vi "Joystick Deadband.vi"(6 "Z Deadband":dbl, 7 "X Y Deadband":dbl, 9 "Z":dbl, 10 "Y":dbl, 11 "X":dbl) -> (1 "Z Out":dbl, 2 "Y Out":dbl, 3 "X Out":dbl)   [LabVIEW 2018]
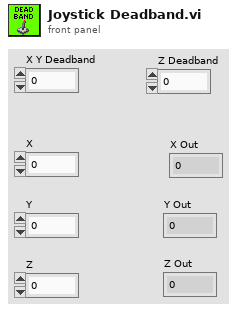
[diagram p1: front panel]
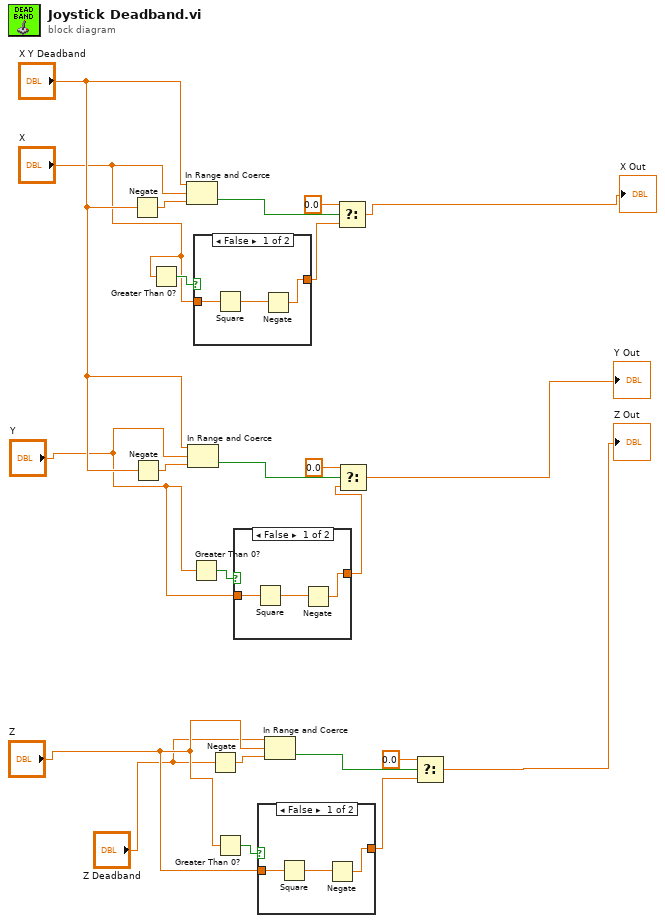
[diagram p0: block diagram]
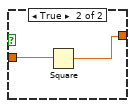
[diagram p2: hidden frame]
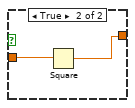
[diagram p3: hidden frame]
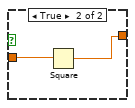
[diagram p4: hidden frame]
diagram:
  n1 = Negate(x="X Y Deadband") -> (-x=w23:dbl)
  n2 = Negate(x="X Y Deadband") -> (-x=w20:dbl)
  n3 = Greater Than 0?(x="X") -> (x > 0?=w10:bool)
  n4 = In Range and Coerce(upper limit="X Y Deadband", x="X", lower limit=w23) -> (In Range?=w22:bool)  [unwired: 1 out]
  n5 = In Range and Coerce(upper limit="X Y Deadband", x="Y", lower limit=w20) -> (In Range?=w19:bool)  [unwired: 1 out]
  n6 = Greater Than 0?(x="Y") -> (x > 0?=w8:bool)
  n7 = case shown="False" w10 {
    tunnel: [w24 w27] -> w11
    tunnel: "X" -> [w26 w28]
    frame False {
      n8 = Square(x=w26) -> (x^2=w25:dbl)
      n9 = Negate(x=w25) -> (-x=w24:dbl)
    }
    frame True {
      n10 = Square(x=w28) -> (x^2=w27:dbl)
    }
  }
  n11 = Negate(x="Z Deadband") -> (-x=w14:dbl)
  n12 = Greater Than 0?(x="Z") -> (x > 0?=w5:bool)
  n13 = case shown="False" w8 {
    tunnel: [w29 w32] -> w6
    tunnel: "Y" -> [w31 w33]
    frame False {
      n14 = Square(x=w31) -> (x^2=w30:dbl)
      n15 = Negate(x=w30) -> (-x=w29:dbl)
    }
    frame True {
      n16 = Square(x=w33) -> (x^2=w32:dbl)
    }
  }
  n17 = case shown="False" w5 {
    tunnel: [w34 w37] -> w4
    tunnel: "Z" -> [w36 w38]
    frame False {
      n18 = Square(x=w36) -> (x^2=w35:dbl)
      n19 = Negate(x=w35) -> (-x=w34:dbl)
    }
    frame True {
      n20 = Square(x=w38) -> (x^2=w37:dbl)
    }
  }
  n21 = In Range and Coerce(upper limit="Z Deadband", x="Z", lower limit=w14) -> (In Range?=w13:bool)  [unwired: 1 out]
  n22 = Select(t=0.0, s=w22, f=w11) -> (s? t:f=→"X Out":dbl)
  n23 = Select(t=0.0, s=w19, f=w6) -> (s? t:f=→"Y Out":dbl)
  n24 = Select(t=0.0, s=w13, f=w4) -> (s? t:f=→"Z Out":dbl)
